vi "DSF.Engine.Framework.Send Base Pointer to Transceivers.vi"(8 "error in (no error)":errorcluster, 9 "engine size":u64, 10 "engine base address":u64 format="%.0x", 11 "Framework in":refnum<class "DSF.Engine.Framework.lvclass">) -> (0 "error out":errorcluster, 3 "Framework out":refnum<class "DSF.Engine.Framework.lvclass">)   [LabVIEW 2017, in "DSF.Engine.lvlib" / "DSF.Engine.Framework.lvclass"]
uses:
  DSF.Engine.Framework.lvclass
  DSF.Engine.Framework.lvclass/DSF.Engine.Framework.ctl
  Plugin/DSF.Engine.Plugin.lvclass/DSF.Engine.Plugin.ctl
  Transceiver/DSF.Engine.Transceiver Thread.lvclass
  Plugin/DSF.Engine.Plugin.lvclass
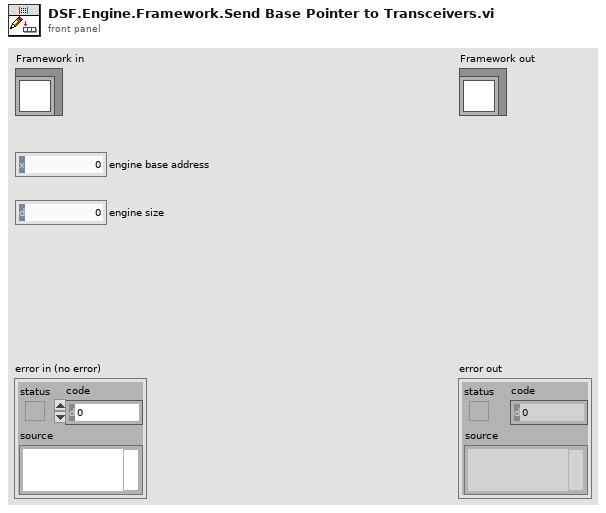
[diagram p1: front panel]
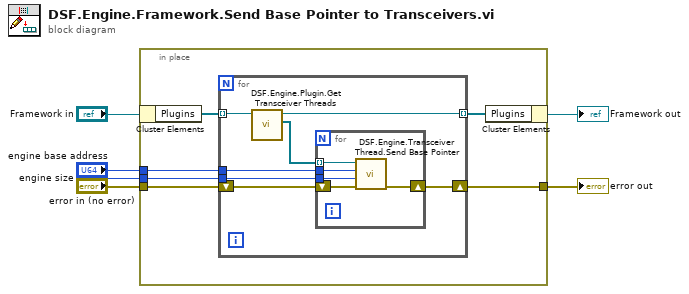
[diagram p0: block diagram]
diagram:
  n1 = in-place {
    in-place-border: "engine base address" -> [w10]
    in-place-border: "engine size" -> [w9]
    in-place-border: "error in (no error)" -> [w8]
    in-place-border: [w7] -> w1
    n2 = in-place-cluster #1("Framework in") -> ("Plugins"=w12:refnum<class "DSF.Engine.Plugin.lvclass">[])
    n3 = for {
      tunnel: w12 -> [w19] mode=indexing
      tunnel: [w18] -> w11 mode=indexing
      tunnel: w10 -> [w16]
      tunnel: w9 -> [w15]
      shift-right: [w14] -> w7
      shift-left: w8 -> [w13]
      n4 = call "DSF.Engine.Plugin.Get Transceiver Threads.vi"("Plugin in"=w19) -> ("Transceiver Threads"=w17:refnum<class "DSF.Engine.Interface.Transceiver.lvclass">[], "Plugin out"=w18:refnum<class "DSF.Engine.Plugin.lvclass">)  [unwired: 9 in]
      n5 = for {
        tunnel: w17 -> [w24] mode=indexing
        shift-right: [w23] -> w14
        shift-left: w13 -> [w22]
        tunnel: w16 -> [w21]
        tunnel: w15 -> [w20]
        n6 = call "DSF.Engine.Transceiver Thread.Send Base Pointer.vi"("error in (no error)"=w22, "engine size"=w20, "engine base address"=w21, "Transceiver Interface in"=w24) -> ("error out"=w23:errorcluster)  [unwired: 6 in, 1 out]
      }
    }
    n7 = in-place-cluster #1("Plugins"=w11) -> (→"Framework out":refnum<class "DSF.Engine.Framework.lvclass">)
  }
  "error out" <- w1
